vi "Mixer.WaitForReady.vi"(1 "Timeout (s)":dbl) -> (0 "ready":bool)   [LabVIEW 2020]
uses:
  SubVIs/Mixer.Globals.vi
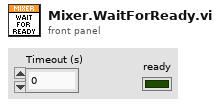
[diagram p1: front panel]
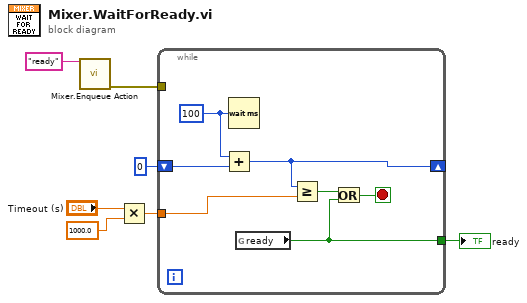
[diagram p0: block diagram]
diagram:
  n1 = call "Mixer.Enqueue Action.vi"("action"="ready") -> ("error out"=w6:errorcluster)  [unwired: 14 in]
  n2 = Multiply(x="Timeout (s)", y=1000.0) -> (x*y=w2:dbl)
  n3 = while {
    tunnel: w6 -> [_]
    shift-right: [w12] -> _
    shift-left: 0 -> [w13]
    tunnel: w2 -> [w11]
    tunnel: [w8] -> w1
    stop <- w9 stop-if-true
    w14 = u32 100 ("milliseconds to wait")
    n4 = Add(x=w14, y=w13) -> (x+y=w12:u32)
    n5 = Wait (ms)(milliseconds to wait=w14) -> ()  [unwired: 1 out]
    n6 = global read "Mixer.Globals.vi" "ready"() -> (w8:bool)
    n7 = Greater Or Equal?(x=w12, y=w11) -> (x >= y?=w10:bool)
    n8 = Or(x=w10, y=w8) -> (x .or. y?=w9:bool)
  }
  "ready" <- w1
